vi "Read LCR Meter.lvclass.vi"(11 "LCR-Measurement in":refnum<class "OTP_LCR_Meas.lvclass">) -> (2 "LCR Meter.lvclass":refnum<class "LCR Meter.lvclass">, 3 "LCR-Measurement out":refnum<class "OTP_LCR_Meas.lvclass">)   [LabVIEW 2020, in "OTP_LCR_Meas.lvclass"]
uses:
  OTP_LCR_Meas.lvclass
  Instruments/LCR Meter/LCR Meter.lvclass
  OTP_LCR_Meas.lvclass/OTP_LCR_Meas.ctl
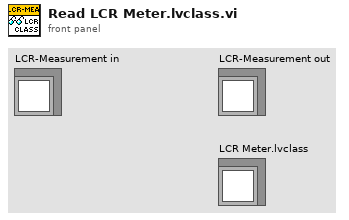
[diagram p1: front panel]
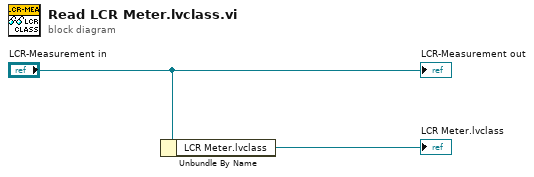
[diagram p0: block diagram]
diagram:
  n1 = Unbundle By Name("LCR-Measurement in") -> ("LCR Meter.lvclass"=→"LCR Meter.lvclass":refnum<class "LCR Meter.lvclass">)
  "LCR-Measurement out" <- "LCR-Measurement in"
